vi "Splashy.GetProtectedEvents.vi"(8 "error in (no error)":errorcluster, 11 "Splashy":refnum<class "Splashy.lvclass">) -> (0 "error out":errorcluster, 2 "Protected Events":T1, 3 "Splashy out":refnum<class "Splashy.lvclass">)   [LabVIEW 2020, in "Splashy.lvclass"]
uses:
  Splashy.lvclass
  Typedefs/ProtectedEvents--Cluster.ctl
  Typedefs/DisplayMessage--Cluster.ctl
  Splashy.lvclass/Splashy.ctl
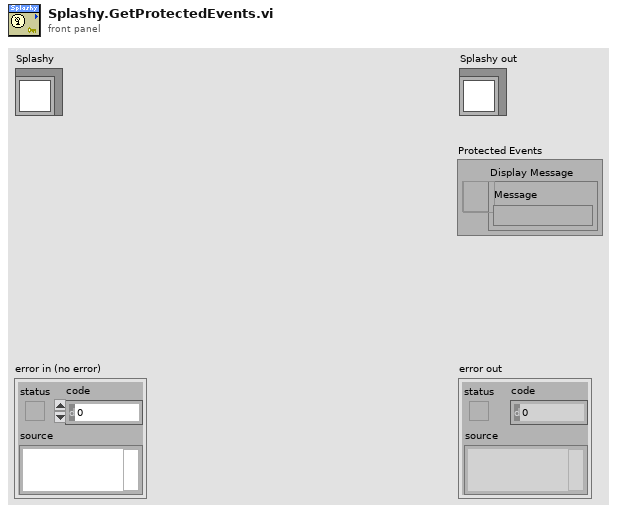
[diagram p1: front panel]
types:
  T1 = typedef "Splashy.lvclass/ProtectedEvents--Cluster.ctl" = cluster{"Display Message":T2}
  T2 = typedef "Splashy.lvclass/DisplayMessage--Cluster.ctl" = refnum<user-event>
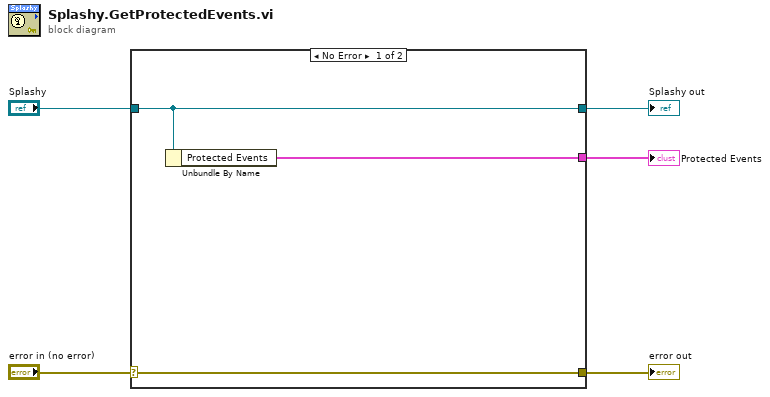
[diagram p0: block diagram]
diagram:
  n1 = case shown="No Error" "error in (no error)" {
    selector: "error in (no error)" -> [w8 w10]
    tunnel: [w8 w10] -> w4
    tunnel: [w7 w9] -> w2
    tunnel: "Splashy" -> [w7 w9]
    tunnel: [w6 _] -> w1
    frame No Error {
      n2 = Unbundle By Name(w7) -> ("Protected Events"=w6:T1)
    }
    frame Error {
    }
  }
  "error out" <- w4
  "Splashy out" <- w2
  "Protected Events" <- w1
